vi "Main.vi"(8 "error in (no error)":errorcluster, 11 "ModuleAdmin":refnum<class "ModuleAdmin.lvclass">) -> ()   [LabVIEW 2018, in "FgenPlugins.lvlib"]
uses:
  FgenPlugins.lvlib
  <userlib>/NIST/ModuleAdminLib/ModuleAdmin/ModuleAdmin.lvclass
  C:/Program Files (x86)/National Instruments/LabVIEW 2018/user.lib/NIST/ModuleAdminLib/ModuleAdminBase/ModuleAdminBase.lvclass
  FgenShared/clStopArgument.ctl
  FgenPluginBaseClass/FgenPluginsBase.lvclass
  C:/Program Files (x86)/National Instruments/LabVIEW 2018/user.lib/NIST/BaseClasses/BasePlugin_class/BasePlugin.lvclass
  <userlib>/NIST/ModuleAdminLib/ModuleAdmin/ModuleAdmin.lvclass/ModuleAdmin.ctl
  FgenPluginBaseClass/FgenPluginsBase.lvclass/FgenPluginsBase.ctl
  MemberClasses/FunctionBaseClass/FunctionBase.lvclass/FunctionBase.ctl
  TypeDefs/clTriggers.ctl
  TypeDefs/Trigger.ctl
  TypeDefs/TriggerType.ctl
  <userlib>/NIST/BaseClasses/BasePlugin_class/BasePlugin.lvclass/BasePlugin.ctl
  TypeDefs/InitOptions.ctl
  TypeDefs/Channels.ctl
  TypeDefs/Channel.ctl
  <vilib>/Utility/error.llb/DialogType.ctl
  <userlib>/NIST/ModuleAdminLib/ModuleAdmin/Accessors/Read ShowPanel_.vi
  <userlib>/NIST/ModuleAdminLib/ModuleAdmin/Accessors/Write ShowPanel_.vi
  FgenPluginBaseClass/Accessors/Read FunctionClass.vi
  FgenPluginBaseClass/Accessors/Write FunctionClass.vi
  MemberClasses/FunctionBaseClass/Accessors/Write Waveforms.vi
  MemberClasses/FunctionBaseClass/Accessors/Read Waveforms.vi
  FgenPluginBaseClass/Accessors/Write Triggers.vi
  FgenPluginBaseClass/Read Triggers.vi
  <userlib>/NIST/BaseClasses/BasePlugin_class/Accessors/Read PluginIniFilePath.vi
  <userlib>/NIST/ModuleAdminLib/ModuleAdmin/Accessors/Read CloneRegRef.vi
  <extravilib>/ChannelInstances/Tag-bool/Read With Abort.vi
  <extravilib>/ChannelInstances/Tag-bool/Write With Abort.vi
  <extravilib>/ChannelInstances/Tag-bool/Instantiate.vi
  <extravilib>/ChannelInstances/Tag-bool/EndpointRead.vi
  <vilib>/Utility/error.llb/Error Cluster From Error Code.vi
  <extravilib>/ChannelInstances/Tag-bool/Endpoint.vi
  <vilib>/ErrorRing/Error Ring.xnode
  MemberClasses/FunctionBaseClass/FunctionBase.lvclass
  <userlib>/NIST/ModuleAdminLib/CloneRegistration/CloneRegistration.lvclass
  FgenShared/FgenShared.lvlib
  <userlib>/NIST/BaseClasses/Object_class/BaseObject.lvclass
  <userlib>/NIST/ModuleAdminLib/ModuleAdmin.lvlib
  <extravilib>/ChannelInstances/Tag-bool.lvlib
panel:
  out "Class Name":string
  out "INI File Name":string
  out "error out":errorcluster
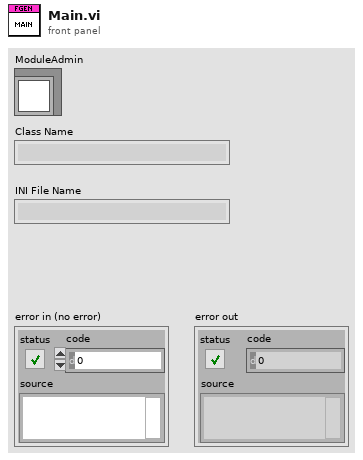
[diagram p1: front panel]
types:
  T1 = typedef "FgenShared.lvlib/clRequestEvents.ctl" = cluster{"StopRequest":refnum<user-event>, "PathToINI":refnum<user-event>, " LoadPlugin":refnum<user-event>, "ShowPanel":refnum<user-event>, "Initialize":refnum<user-event>, "GetChannels":refnum<user-event>, "SetChannels":refnum<user-event>, "Abort":refnum<user-event>, "Initiate":refnum<user-event>, "ConfigDlg":refnum<user-event>, "GetFunction":refnum<user-event>, "SetFunction":refnum<user-event>, "ConfigFunction":refnum<user-event>, "GetWfrm":refnum<user-event>, "SetWfrm":refnum<user-event>, "GetTriggers":refnum<user-event>, "SetTriggers":refnum<user-event>, "ConfigTriggers":refnum<user-event>, "Close":refnum<user-event>, "GetFunctionParams":refnum<user-event>, "SetFunctionParams":refnum<user-event>, "GetFunctionArbs":refnum<user-event>, "SetFunctionArbs":refnum<user-event>, "GetFunctionSampleRate":refnum<user-event>, "SetFunctionSampleRate":refnum<user-event>}
  T2 = typedef "FgenShared.lvlib/clBroadcastEvents.ctl" = cluster{"DidInit":refnum<user-event>, "StatusUpdate":refnum<user-event>, "ErrorReport":refnum<user-event>, "DidStop":refnum<user-event>, "PathToINI":refnum<user-event>, "Channels":refnum<user-event>, "Function":refnum<user-event>, "Waveforms":refnum<user-event>, "Triggers":refnum<user-event>, "FunctionParams":refnum<user-event>, "FunctionArbs":refnum<user-event>, "FunctionSampleRate":refnum<user-event>}
  T3 = typedef "FgenShared.lvlib/clStopArgument.ctl" = cluster{"Exit via Stop Module Req?":bool, "Wait for Module to stop?":bool, "ModuleAdmin":refnum<class "ModuleAdmin.lvclass">}
  T4 = enum32{"Invalid", "Standard", "Closed", "Hidden", "Minimized", "Maximized"}
  T5 = typedef "FgenPlugins.lvlib/clTriggers.ctl" = cluster{"Count":i32, "Triggers":T6[]}
  T6 = typedef "FgenPlugins.lvlib/Trigger.ctl" = cluster{"Source":string, "Slope":enum16{"Positive", "Negative", "Either"}, "Threshold":dbl, "Delay":dbl, "TriggerType":T7}
  T7 = typedef "FgenPlugins.lvlib/TriggerType.ctl" = enum16{"None", "Start", "Stop", "Hold", "Resume", "Advance"}
  T8 = typedef "FgenPlugins.lvlib/InitOptions.ctl" = cluster{"IDQuery":bool, "Reset":bool}
  T9 = typedef "FgenPlugins.lvlib/Channels.ctl" = cluster{"Count":u16, "Channel":T10[]}
  T10 = typedef "FgenPlugins.lvlib/Channel.ctl" = cluster{"Name":string, "Enabled":bool, "Operation":enum16{"Continuous", "Burst"}, "Impedance (50)":dbl, "Handle":string, "Connected":bool, "Mode (Function)":enum16{"Function", "Arbitrary", "Sequence"}}
  T11 = typedef "Tag-bool.lvlib/))Channel.ctl" = refnum<queue>
  T12 = typedef "DialogType.ctl" = u16
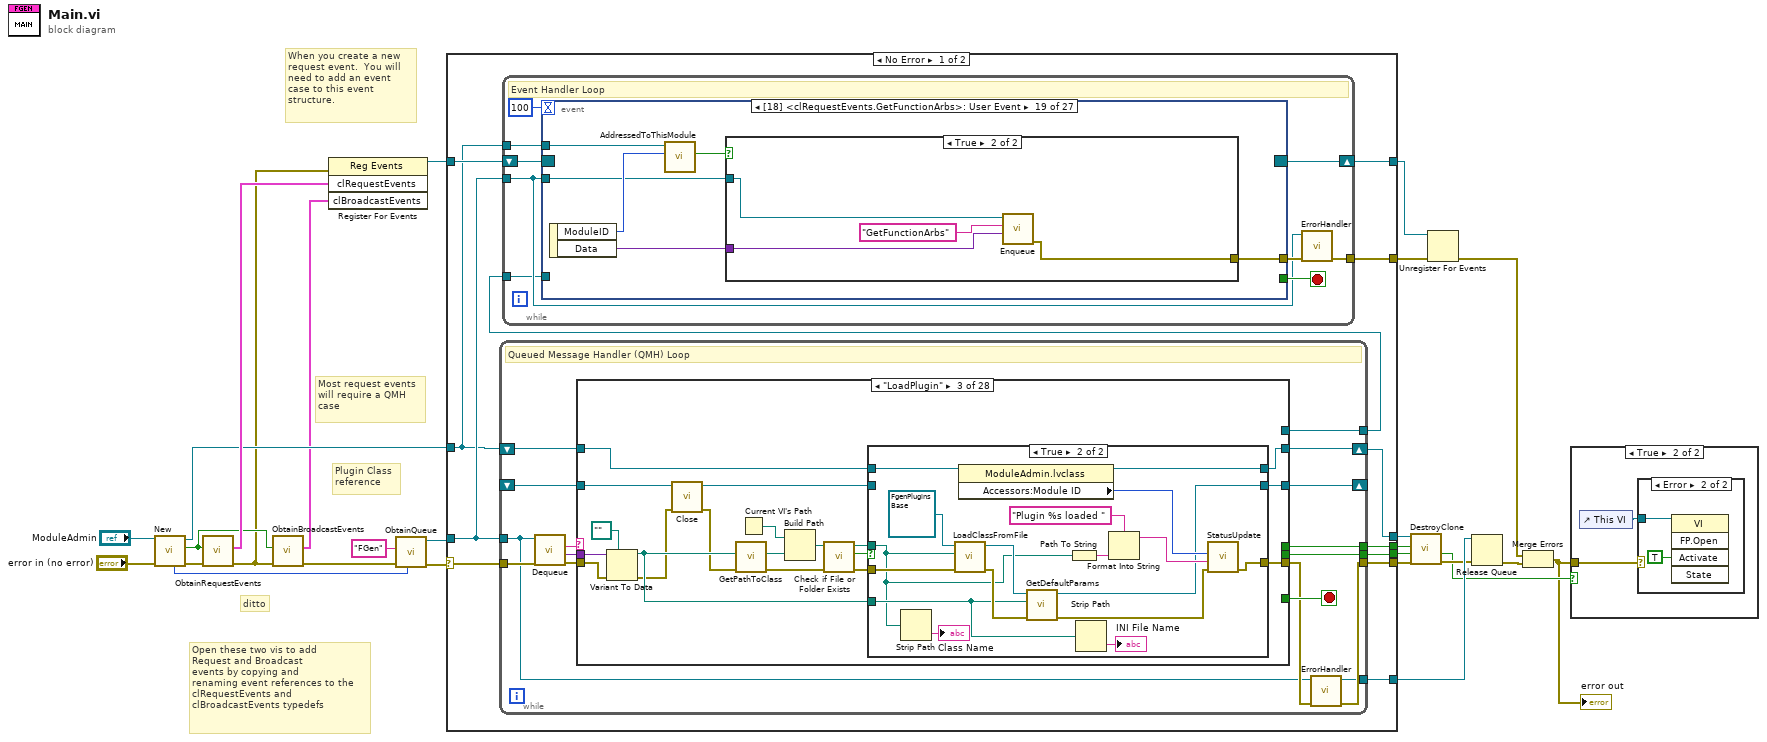
[diagram p0: block diagram]
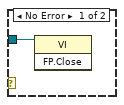
[diagram p3: hidden frame]
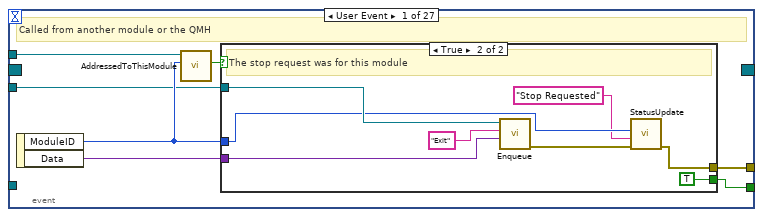
[diagram p4: hidden frame]
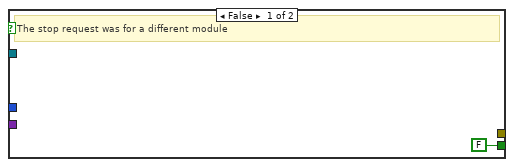
[diagram p5: hidden frame]
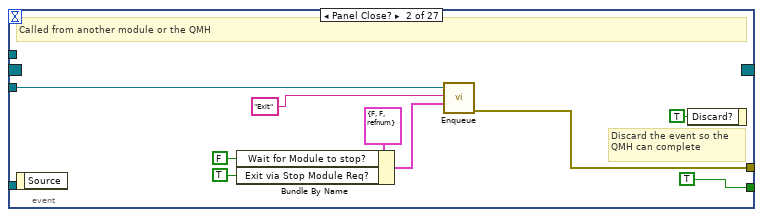
[diagram p6: hidden frame]
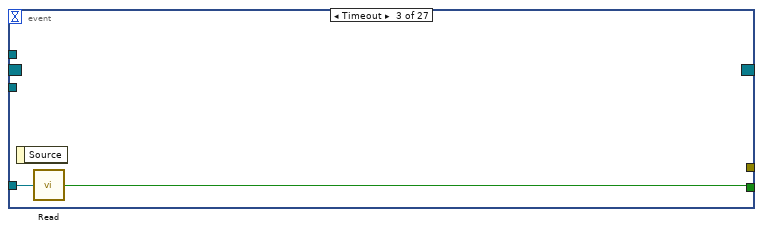
[diagram p7: hidden frame]
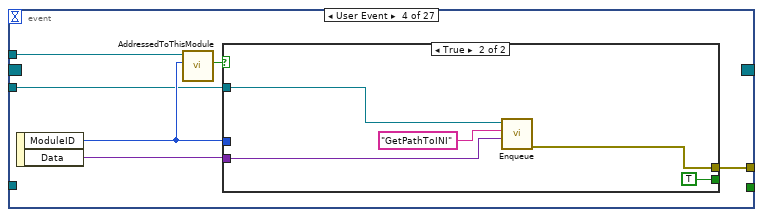
[diagram p8: hidden frame]
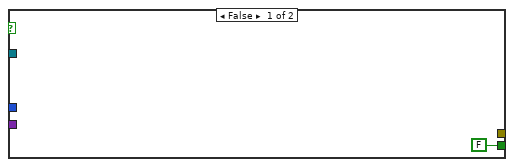
[diagram p9: hidden frame]
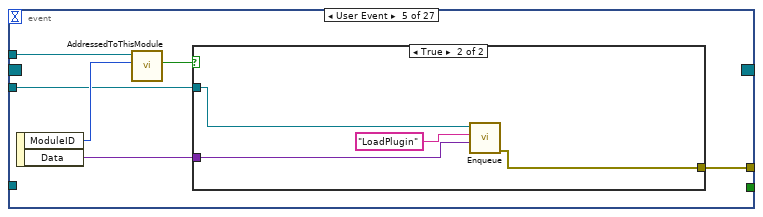
[diagram p10: hidden frame]
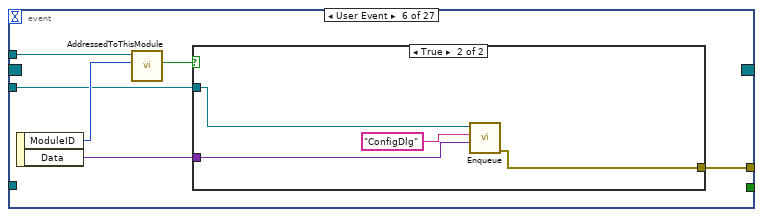
[diagram p12: hidden frame]
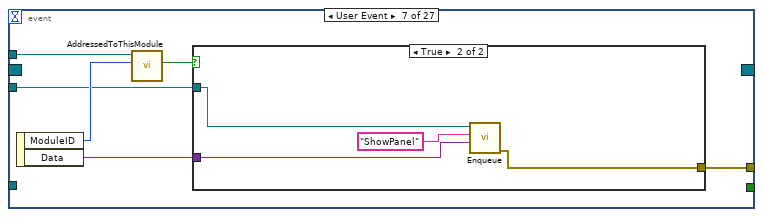
[diagram p14: hidden frame]
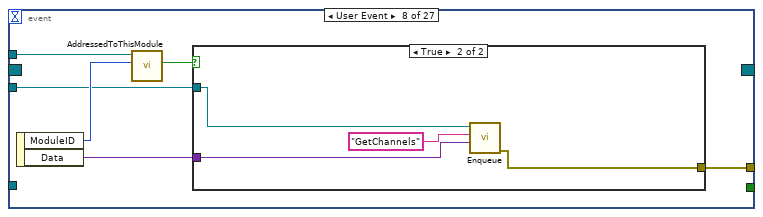
[diagram p16: hidden frame]
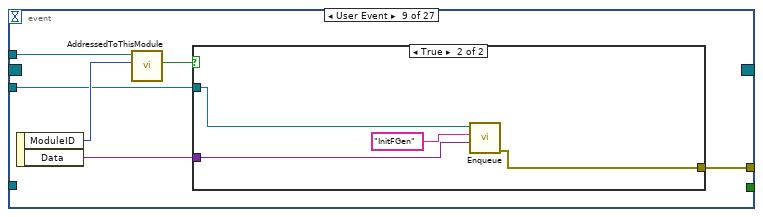
[diagram p18: hidden frame]
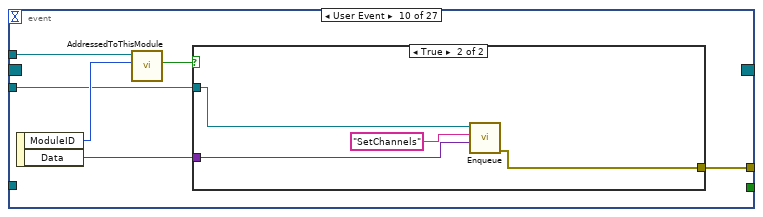
[diagram p20: hidden frame]
diagram:
  # "Plugin Class\nreference"
  # "Open these two vis to add\nRequest and Broadcast \nevents by copying and \nrenaming event references to the \nclRequestEvents and \nclBroadcastEvents typedefs"
  # "ditto"
  # "Most request events\nwill require a QMH\ncase"
  # "When you create a new request event.  You will need to add an event case to this event structure."
  n1 = call <userlib>:"New.vi"("error in (no error)"="error in (no error)", "ModuleAdmin"="ModuleAdmin") -> ("error out"=w24:errorcluster, "First?"=w17:bool, "ModuleAdmin"=w20:refnum<class "ModuleAdmin.lvclass">, "Module ID"=w6:i32)  [unwired: 6 in]
  n2 = call "ObtainRequestEvents.vi"("error in (no error)"=w24, "CreateNew (F)"=w17) -> ("error out"=w16:errorcluster, "clRequestEvents"=w23:T1)  [unwired: 8 in]
  n3 = call "ObtainBroadcastEvents.vi"("error in (no error)"=w16, "CreateNew? (F)"=w17) -> ("error out"=w18:errorcluster, "clBroadcastEvents"=w15:T2)  [unwired: 8 in]
  n4 = register-events(error in=w16, w23, w15) -> (reference out=w14:refnum<event-registration>)  [unwired: 1 in, 1 out]
  n5 = call "ObtainQueue.vi"("Module ID"=w6, "error in (no error)"=w18, "ModuleName"="FGen") -> ("error out"=w22:errorcluster, "MessageQueue"=w21:refnum<queue>)  [unwired: 7 in]
  n6 = case shown="No Error" w22 {
    selector: w22 -> [w38 w761]
    tunnel: w21 -> [w36 w758]
    tunnel: w20 -> [w33 w759]
    tunnel: [w37 w753] -> w13
    tunnel: [w35 w758] -> w19
    tunnel: w14 -> [w34 w754]
    tunnel: [w32 w757] -> w11
    tunnel: [w31 _] -> w10
    tunnel: [w30 _] -> w9
    tunnel: [w29 w753] -> w4
    tunnel: [w27 w754] -> w3
    frame No Error {
      n7 = while {
        tunnel: w36 -> [w318]
        tunnel: w38 -> [w331]
        tunnel: [w324] -> w37
        tunnel: [w317] -> w35
        tunnel: [w326] -> w31
        tunnel: [w325] -> w30
        shift-right: [w322] -> _
        shift-left: _ -> [w321]
        shift-right: [w320] -> w32
        shift-left: w33 -> [w327]
        tunnel: [w319] -> w28
        stop <- w332 stop-if-true
        # "Queued Message Handler (QMH) Loop"
        n8 = call "Dequeue.vi"("error in (no error)"=w331, "MessageQueue"=w318) -> ("error out"=w330:errorcluster, "Message Data"=w328:variant, "Message"=w329:string)  [unwired: 6 in, 1 out]
        n9 = case shown="\"LoadPlugin\"" w329 {
          selector: w329 -> [_ _ _ _ _ _ _ _ _ _ _ _ _ _ _ _ _ _ _ _ _ _ _ _ _ _ _ w741]
          tunnel: [_ _ _ _ _ _ _ _ _ _ _ _ _ _ _ _ _ _ _ _ _ _ _ _ _ w719 _ _] -> w332
          tunnel: w327 -> [w353 w370 w381 w430 w444 w451 w481 w499 w510 w521 w536 w551 w566 w584 w595 w607 w617 w624 w633 w650 w665 w672 w680 w689 w700 w713 w722 w744]
          tunnel: [w342 w363 w382 w424 w442 w447 w472 w494 w501 w515 w533 w548 w563 w573 w593 w598 w611 w619 w634 w643 w656 w666 w677 w686 w701 w718 w723 w740] -> w323
          tunnel: w330 -> [_ w373 w390 w429 w438 w457 w479 w497 w508 w519 w527 w542 w557 w580 w591 w606 w613 w625 w629 w652 w662 w674 w682 w691 w695 w709 w731 _]
          tunnel: w328 -> [_ w372 w392 _ _ w452 _ _ _ _ w529 w544 w559 w579 _ w605 _ _ _ w651 w663 _ _ _ _ w717 w730 _]
          tunnel: [_ _ _ _ _ _ _ _ _ _ _ _ _ _ _ _ _ _ _ _ _ _ _ _ _ w715 _ _] -> w326
          tunnel: [_ _ _ _ _ _ _ _ _ _ _ _ _ _ _ _ _ _ _ _ _ _ _ _ _ w714 _ _] -> w325
          tunnel: [refnum<class "FgenPluginsBase.lvclass"> refnum ("MyPlugins.lvlib:MyPluginsBase.lvclass") w362 w380 w427 w437 w446 w471 w493 w506 w517 w523 w538 w553 w572 w587 w596 w609 w623 w630 w636 w660 w669 w681 w690 w698 w712 w721 w738] -> w322
          tunnel: w321 -> [_ w362 w377 w428 w439 w459 w480 w498 w509 w520 w531 w546 w561 w582 w592 w608 w615 w626 w632 w649 w661 w673 w683 w692 w699 w711 w721 w738]
          tunnel: [w333 w369 w378 w426 w443 w445 w476 w496 w507 w518 w535 w550 w565 w583 w585 w597 w610 w622 w627 w642 w655 w668 w679 w688 w697 w707 w720 w737] -> w320
          tunnel: [_ _ _ _ _ _ _ _ _ _ _ _ _ _ _ _ _ _ _ _ _ _ _ _ _ w702 _ _] -> w319
          frame "Initialize" {
            # "Initialize is always called after ObtainQueue.vi is run"
            n10 = property class="ModuleAdmin.lvclass"(reference=w353) -> (reference out=w339:refnum<class "ModuleAdmin.lvclass">, error out=w350:errorcluster, "Accessors:Module ID"=w341:i32, "Accessors:ShowPanel_"=w336:bool, "Accessors:External Launch"=w335:bool, "Accessors:ModuleName"=w337:string)  [unwired: 1 in]
            n11 = Compound Arithmetic op=OR(w336, invert w335) -> (w334:bool)
            n12 = Select(t=T4."Standard" ("Front Panel Window:State"), s=w334, f=T4."Hidden" ("Front Panel Window:State")) -> (s? t:f=w346:T4)
            n13 = invoke class="VI" method="FP.Open"(error in=w350, "State"=w346) -> (error out=w349:errorcluster)  [unwired: 3 in, 4 out]
            n14 = call <userlib>:"ModuleName.vi"("Name"=w337, "ModuleID"=w341) -> ("ModuleName"=w345:string)  [unwired: 9 in]
            n15 = property class="VI"(error in=w349, "Front Panel.Title"=w345) -> (reference out=w352:refnum<vi>, error out=w351:errorcluster)  [unwired: 1 in]
            n16 = invoke class="VI" method="FP.Center"(reference=w352, error in=w351) -> (error out=w340:errorcluster)  [unwired: 1 in, 2 out]
            n17 = case shown="True" w335 {
              tunnel: [w354 w360] -> w343
              tunnel: [w355 w357] -> w333
              tunnel: w340 -> [w354 w359]
              tunnel: w339 -> [w355 w356]
              frame False {
              }
              frame True {
                n18 = call <userlib>:"WaitOnModuleSync.vi"("error in (no error)"=w359, "ModuleAdmin"=w356) -> ("error out"=w361:errorcluster, "ModuleAdmin"=w358:refnum<class "ModuleAdmin.lvclass">)  [unwired: 8 in]
                n19 = call <userlib>:"WaitOnEventSync.vi"("error in (no error)"=w361, "ModuleAdmin"=w358) -> ("error out"=w360:errorcluster, "ModuleAdmin"=w357:refnum<class "ModuleAdmin.lvclass">)  [unwired: 8 in]
              }
            }
            n20 = call "DidInit.vi"("Init?"=TRUE, "error in (no error)"=w343, "ModuleAdmin"=w333) -> ("error out"=w342:errorcluster)  [unwired: 8 in]
          }
          frame "ShowPanel" {
            n21 = Variant To Data(error in=w373, type=TRUE, Variant=w372) -> (data=w365:bool, error out=w368:errorcluster)
            n22 = Select(t=T4."Standard" ("Front Panel Window:State"), s=w365, f=T4."Hidden" ("Front Panel Window:State")) -> (s? t:f=w364:T4)
            n23 = property class="VI"(error in=w368, "FP.State"=w364) -> (error out=w363:errorcluster)  [unwired: 1 in, 1 out]
            n24 = property class="ModuleAdmin.lvclass"(reference=w370, "Accessors:ShowPanel_"=w365) -> (reference out=w369:refnum<class "ModuleAdmin.lvclass">)  [unwired: 1 in, 1 out]
          }
          frame "LoadPlugin" {
            n25 = Variant To Data(error in=w390, type=path "", Variant=w392) -> (data=w379:path, error out=w375:errorcluster)
            n26 = call-dynamic "Close.vi"("error in (no error)"=w375, "FgenPluginsBase in"=w377) -> ("error out"=w374:errorcluster, "FgenPluginsBase out"=w376:refnum<class "FgenPluginsBase.lvclass">)  [unwired: 8 in]
            n27 = call <userlib>:"GetPathToClass.vi"("error in (no error)"=w374, "configuration file path"=w379) -> ("error IO"=w386:errorcluster, "PathToClass"=w389:path)  [unwired: 8 in]
            n28 = Current VI's Path() -> (path=w388:path)
            n29 = Build Path(base path=w388, name or relative path=w389) -> (appended path=w387:path)
            n30 = call <vilib>:"Check if File or Folder Exists.vi"("error in (no error)"=w386, "path"=w387) -> ("error out"=w383:errorcluster, "file or folder exists?"=w385:bool, "dup path"=w384:path)  [unwired: 7 in]
            n31 = case shown="True" w385 {
              tunnel: w384 -> [w396 w406]
              tunnel: w383 -> [_ w421]
              tunnel: [w395 w416] -> w382
              tunnel: w381 -> [w393 w415]
              tunnel: w376 -> [w394 _]
              tunnel: [w394 w410] -> w380
              tunnel: w379 -> [_ w407]
              tunnel: [w393 w413] -> w378
              frame False {
                n32 = Path To String(path=w396) -> (string=w397:string)
                n33 = xnode "Error Ring"("parameter 0"=w397) -> ("error out"=w395:errorcluster)
              }
              frame True {
                n34 = Strip Path(path=w406) -> (name=→"Class Name":string)  [unwired: 1 out]
                n35 = call-dynamic "LoadClassFromFile.vi"("error in (no error)"=w421, "class path"=w406, "reference in"=refnum<class "FgenPluginsBase.lvclass"> refnum ("MyPlugins.lvlib:MyPluginsBase.lvclass")) -> ("error out"=w412:errorcluster, "reference out"=w411:refnum<class "FgenPluginsBase.lvclass">)  [unwired: 7 in]
                n36 = property class="ModuleAdmin.lvclass"(reference=w415) -> (reference out=w413:refnum<class "ModuleAdmin.lvclass">, "Accessors:Module ID"=w414:i32)  [unwired: 1 in, 1 out]
                n37 = call-dynamic "GetDefaultParams.vi"("error in (no error)"=w412, "Path"=w407, "FgenPluginsBase in"=w411) -> ("error out"=w409:errorcluster, "FgenPluginsBase out"=w410:refnum<class "FgenPluginsBase.lvclass">)  [unwired: 7 in]
                n38 = Path To String(path=w406) -> (string=w418:string)
                n39 = Strip Path(path=w407) -> (name=→"INI File Name":string)  [unwired: 1 out]
                n40 = Format Into String(format string="Plugin %s loaded ", w418) -> (resulting string=w417:string)  [unwired: 2 in, 1 out]
                n41 = call "StatusUpdate.vi"("error in (no error)"=w409, "Status"=w417, "ModuleID"=w414) -> ("error out"=w416:errorcluster)  [unwired: 8 in]
              }
            }
          }
          frame "ConfigDlg" {
            n42 = call-dynamic "ConfigDlg.vi"("error in (no error)"=w429, "FgenPluginsBase in"=w428) -> ("error out"=w425:errorcluster, "Changed"=w422:bool, "FgenPluginsBase out"=w427:refnum<class "FgenPluginsBase.lvclass">)  [unwired: 7 in]
            n43 = property class="ModuleAdmin.lvclass"(reference=w430) -> (reference out=w426:refnum<class "ModuleAdmin.lvclass">, "Accessors:Module ID"=w423:i32)  [unwired: 1 in, 1 out]
            n44 = case shown="True" w422 {
              tunnel: w425 -> [w431 w435]
              tunnel: [w431 w434] -> w424
              tunnel: w423 -> [_ w433]
              frame False {
              }
              frame True {
                n45 = call "StatusUpdate.vi"("error in (no error)"=w435, "Status"="Configuration Updated", "ModuleID"=w433) -> ("error out"=w434:errorcluster)  [unwired: 8 in]
              }
            }
          }
          frame "ConfigFunction" {
            n46 = call-dynamic "ConfigFunction.vi"("error in (no error)"=w438, "FgenPluginsBase in"=w439) -> ("error out"=w436:errorcluster, "FgenPluginsBase out"=w437:refnum<class "FgenPluginsBase.lvclass">)  [unwired: 8 in]
            n47 = property class="ModuleAdmin.lvclass"(reference=w444) -> (reference out=w443:refnum<class "ModuleAdmin.lvclass">, "Accessors:Module ID"=w441:i32)  [unwired: 1 in, 1 out]
            n48 = call "StatusUpdate.vi"("error in (no error)"=w436, "Status"="Function Configured", "ModuleID"=w441) -> ("error out"=w442:errorcluster)  [unwired: 8 in]
          }
          frame "SetFunction" {
            n49 = property class="FgenPluginsBase.lvclass"(reference=w459, error in=w457) -> (reference out=w458:refnum<class "FgenPluginsBase.lvclass">, error out=w455:errorcluster, "Accessors:FunctionClass"=w456:refnum<class "FunctionBase.lvclass">)
            n50 = disable-structure shown="Enabled" {
              disable-tunnel: w456 -> [w464 w468]
              disable-tunnel: w455 -> [w463 w467]
              disable-tunnel: [w462 w466] -> w454
              disable-tunnel: [w461 w465] -> w453
              disable-tunnel: w452 -> [w460 w469]
              frame Disabled {
                n51 = call-dynamic "SetConfig.vi"("error in (no error)"=w463, "Variant"=w460, "FunctionBase in"=w464) -> ("error out"=w462:errorcluster, "FunctionBase out"=w461:refnum<class "FunctionBase.lvclass">)  [unwired: 7 in]
              }
              frame Enabled {
                n52 = Variant To Data(error in=w467, type=w468, Variant=w469) -> (data=w465:refnum<class "FunctionBase.lvclass">, error out=w466:errorcluster)
              }
            }
            n53 = property class="FgenPluginsBase.lvclass"(reference=w458, error in=w454, "Accessors:FunctionClass"=w453) -> (reference out=w446:refnum<class "FgenPluginsBase.lvclass">, error out=w448:errorcluster)
            n54 = property class="ModuleAdmin.lvclass"(reference=w451) -> (reference out=w445:refnum<class "ModuleAdmin.lvclass">, "Accessors:Module ID"=w449:i32)  [unwired: 1 in, 1 out]
            n55 = call "StatusUpdate.vi"("error in (no error)"=w448, "Status"="Function Set", "ModuleID"=w449) -> ("error out"=w447:errorcluster)  [unwired: 8 in]
          }
          frame "GetFunction" {
            n56 = property class="FgenPluginsBase.lvclass"(reference=w480, error in=w479) -> (reference out=w471:refnum<class "FgenPluginsBase.lvclass">, error out=w477:errorcluster, "Accessors:FunctionClass"=w478:refnum<class "FunctionBase.lvclass">)
            n57 = property class="ModuleAdmin.lvclass"(reference=w481) -> (reference out=w476:refnum<class "ModuleAdmin.lvclass">, "Accessors:Module ID"=w475:i32)  [unwired: 1 in, 1 out]
            n58 = disable-structure shown="Enabled" {
              disable-tunnel: w478 -> [w485 w487]
              disable-tunnel: w477 -> [w484 w486]
              disable-tunnel: [w483 w487] -> w474
              disable-tunnel: [w482 w486] -> w473
              frame Disabled {
                n59 = call-dynamic "GetConfig.vi"("error in (no error)"=w484, "FunctionBase in"=w485) -> ("error out"=w482:errorcluster, "Config"=w483:variant)  [unwired: 7 in, 1 out]
              }
              frame Enabled {
              }
            }
            n60 = To Variant(anything=w474) -> (Variant=w470:variant)
            n61 = call "Function.vi"("ModuleID"=w475, "error in (no error)"=w473, "Function"=w470) -> ("error out"=w472:errorcluster)  [unwired: 8 in]
          }
          frame "GetFunctionParams" {
            n62 = property class="FgenPluginsBase.lvclass"(reference=w498, error in=w497) -> (reference out=w493:refnum<class "FgenPluginsBase.lvclass">, error out=w490:errorcluster, "Accessors:FunctionClass"=w489:refnum<class "FunctionBase.lvclass">)
            n63 = property class="ModuleAdmin.lvclass"(reference=w499) -> (reference out=w496:refnum<class "ModuleAdmin.lvclass">, "Accessors:Module ID"=w495:i32)  [unwired: 1 in, 1 out]
            n64 = call-dynamic "GetSignalParams.vi"("error in (no error)"=w490, "FunctionBase in"=w489) -> ("error out"=w491:errorcluster, "Params"=w488:variant)  [unwired: 7 in, 1 out]
            n65 = To Variant(anything=w488) -> (Variant=w492:variant)
            n66 = call "FunctionParams.vi"("ModuleID"=w495, "error in (no error)"=w491, "Function"=w492) -> ("error out"=w494:errorcluster)  [unwired: 8 in]
          }
          frame "GetFunctionArbs" {
            n67 = property class="FgenPluginsBase.lvclass"(reference=w509, error in=w508) -> (reference out=w506:refnum<class "FgenPluginsBase.lvclass">, error out=w505:errorcluster, "Accessors:FunctionClass"=w504:refnum<class "FunctionBase.lvclass">)
            n68 = property class="ModuleAdmin.lvclass"(reference=w510) -> (reference out=w507:refnum<class "ModuleAdmin.lvclass">, "Accessors:Module ID"=w503:i32)  [unwired: 1 in, 1 out]
            n69 = call-dynamic "GetFunctionConfig.vi"("error in (no error)"=w505, "FunctionBase In"=w504) -> ("error out"=w502:errorcluster, "FunctionConfig"=w500:variant)  [unwired: 7 in, 1 out]
            n70 = call "FunctionArbs.vi"("ModuleID"=w503, "error in (no error)"=w502, "Function"=w500) -> ("error out"=w501:errorcluster)  [unwired: 8 in]
          }
          frame "GetFunctionSampleRate" {
            n71 = property class="FgenPluginsBase.lvclass"(reference=w520, error in=w519) -> (reference out=w517:refnum<class "FgenPluginsBase.lvclass">, error out=w514:errorcluster, "Accessors:FunctionClass"=w513:refnum<class "FunctionBase.lvclass">)
            n72 = property class="ModuleAdmin.lvclass"(reference=w521) -> (reference out=w518:refnum<class "ModuleAdmin.lvclass">, "Accessors:Module ID"=w516:i32)  [unwired: 1 in, 1 out]
            n73 = call-dynamic "GetFunctionSampleRate.vi"("error in (no error)"=w514, "FunctionBase in"=w513) -> ("error out"=w511:errorcluster, "SampleRate"=w512:variant)  [unwired: 7 in, 1 out]
            n74 = call "FunctionSampleRate.vi"("ModuleID"=w516, "error in (no error)"=w511, "SampleRate"=w512) -> ("error out"=w515:errorcluster)  [unwired: 8 in]
          }
          frame "SetFunctionParams" {
            n75 = property class="FgenPluginsBase.lvclass"(reference=w531, error in=w527) -> (reference out=w528:refnum<class "FgenPluginsBase.lvclass">, error out=w526:errorcluster, "Accessors:FunctionClass"=w530:refnum<class "FunctionBase.lvclass">)
            n76 = call-dynamic "SetSignalParams.vi"("error in (no error)"=w526, "Variant"=w529, "FunctionBase in"=w530) -> ("error out"=w524:errorcluster, "FunctionBase out"=w525:refnum<class "FunctionBase.lvclass">)  [unwired: 7 in]
            n77 = property class="FgenPluginsBase.lvclass"(reference=w528, error in=w524, "Accessors:FunctionClass"=w525) -> (reference out=w523:refnum<class "FgenPluginsBase.lvclass">, error out=w522:errorcluster)
            n78 = property class="ModuleAdmin.lvclass"(reference=w536) -> (reference out=w535:refnum<class "ModuleAdmin.lvclass">, "Accessors:Module ID"=w534:i32)  [unwired: 1 in, 1 out]
            n79 = call "StatusUpdate.vi"("error in (no error)"=w522, "Status"="FunctionParams Set", "ModuleID"=w534) -> ("error out"=w533:errorcluster)  [unwired: 8 in]
          }
          frame "SetFunctionArbs" {
            n80 = property class="FgenPluginsBase.lvclass"(reference=w546, error in=w542) -> (reference out=w543:refnum<class "FgenPluginsBase.lvclass">, error out=w541:errorcluster, "Accessors:FunctionClass"=w545:refnum<class "FunctionBase.lvclass">)
            n81 = call-dynamic "SetFunctionArbs.vi"("error in (no error)"=w541, "Variant"=w544, "FunctionBase in"=w545) -> ("error out"=w539:errorcluster, "FunctionBase out"=w540:refnum<class "FunctionBase.lvclass">)  [unwired: 7 in]
            n82 = property class="FgenPluginsBase.lvclass"(reference=w543, error in=w539, "Accessors:FunctionClass"=w540) -> (reference out=w538:refnum<class "FgenPluginsBase.lvclass">, error out=w537:errorcluster)
            n83 = property class="ModuleAdmin.lvclass"(reference=w551) -> (reference out=w550:refnum<class "ModuleAdmin.lvclass">, "Accessors:Module ID"=w549:i32)  [unwired: 1 in, 1 out]
            n84 = call "StatusUpdate.vi"("error in (no error)"=w537, "Status"="FunctionConfig Set", "ModuleID"=w549) -> ("error out"=w548:errorcluster)  [unwired: 8 in]
          }
          frame "SetFunctionSampleRate" {
            n85 = property class="FgenPluginsBase.lvclass"(reference=w561, error in=w557) -> (reference out=w558:refnum<class "FgenPluginsBase.lvclass">, error out=w556:errorcluster, "Accessors:FunctionClass"=w560:refnum<class "FunctionBase.lvclass">)
            n86 = call-dynamic "SetFunctionSampleRate.vi"("error in (no error)"=w556, "SampleRate"=w559, "FunctionBase in"=w560) -> ("error out"=w554:errorcluster, "FunctionBase out"=w555:refnum<class "FunctionBase.lvclass">)  [unwired: 7 in]
            n87 = property class="FgenPluginsBase.lvclass"(reference=w558, error in=w554, "Accessors:FunctionClass"=w555) -> (reference out=w553:refnum<class "FgenPluginsBase.lvclass">, error out=w552:errorcluster)
            n88 = property class="ModuleAdmin.lvclass"(reference=w566) -> (reference out=w565:refnum<class "ModuleAdmin.lvclass">, "Accessors:Module ID"=w564:i32)  [unwired: 1 in, 1 out]
            n89 = call "StatusUpdate.vi"("error in (no error)"=w552, "Status"="FunctionSampleRate Set", "ModuleID"=w564) -> ("error out"=w563:errorcluster)  [unwired: 8 in]
          }
          frame "SetWfrm" {
            n90 = Variant To Data(error in=w580, type=waveform(dbl)[] [] ("Waveforms"), Variant=w579) -> (data=w577:waveform(dbl)[], error out=w576:errorcluster)
            n91 = property class="FgenPluginsBase.lvclass"(reference=w582, error in=w576) -> (reference out=w568:refnum<class "FgenPluginsBase.lvclass">, error out=w575:errorcluster, "Accessors:FunctionClass"=w581:refnum<class "FunctionBase.lvclass">)
            n92 = property class="FunctionBase.lvclass"(reference=w581, error in=w575, "Accessors:Waveforms"=w577) -> (reference out=w571:refnum<class "FunctionBase.lvclass">, error out=w569:errorcluster)
            n93 = property class="FgenPluginsBase.lvclass"(reference=w568, error in=w569, "Accessors:FunctionClass"=w571) -> (reference out=w572:refnum<class "FgenPluginsBase.lvclass">, error out=w567:errorcluster)
            n94 = property class="ModuleAdmin.lvclass"(reference=w584) -> (reference out=w583:refnum<class "ModuleAdmin.lvclass">, "Accessors:Module ID"=w570:i32)  [unwired: 1 in, 1 out]
            n95 = call "StatusUpdate.vi"("error in (no error)"=w567, "Status"="Waveforms Set", "ModuleID"=w570) -> ("error out"=w573:errorcluster)  [unwired: 8 in]
          }
          frame "GetWfrm" {
            n96 = property class="FgenPluginsBase.lvclass"(reference=w592, error in=w591) -> (reference out=w587:refnum<class "FgenPluginsBase.lvclass">, error out=w586:errorcluster, "Accessors:FunctionClass"=w590:refnum<class "FunctionBase.lvclass">)
            n97 = property class="FunctionBase.lvclass"(reference=w590, error in=w586) -> (error out=w588:errorcluster, "Accessors:Waveforms"=w589:waveform(dbl)[])  [unwired: 1 out]
            n98 = property class="ModuleAdmin.lvclass"(reference=w595) -> (reference out=w585:refnum<class "ModuleAdmin.lvclass">, "Accessors:Module ID"=w594:i32)  [unwired: 1 in, 1 out]
            n99 = call "Waveforms.vi"("ModuleID"=w594, "error in (no error)"=w588, "Waveforms"=w589) -> ("error out"=w593:errorcluster)  [unwired: 8 in]
          }
          frame "SetTriggers" {
            n100 = Variant To Data(error in=w606, type=T5 {"Count"=0, "Triggers"=[]} ("Triggers"), Variant=w605) -> (data=w603:T5, error out=w602:errorcluster)
            n101 = property class="FgenPluginsBase.lvclass"(reference=w608, error in=w602, "Accessors:Triggers"=w603) -> (reference out=w596:refnum<class "FgenPluginsBase.lvclass">, error out=w599:errorcluster)
            n102 = property class="ModuleAdmin.lvclass"(reference=w607) -> (reference out=w597:refnum<class "ModuleAdmin.lvclass">, "Accessors:Module ID"=w600:i32)  [unwired: 1 in, 1 out]
            n103 = call "StatusUpdate.vi"("error in (no error)"=w599, "Status"="Triggers Updated", "ModuleID"=w600) -> ("error out"=w598:errorcluster)  [unwired: 8 in]
          }
          frame "GetTriggers" {
            n104 = property class="ModuleAdmin.lvclass"(reference=w617) -> (reference out=w610:refnum<class "ModuleAdmin.lvclass">, "Accessors:Module ID"=w616:i32)  [unwired: 1 in, 1 out]
            n105 = property class="FgenPluginsBase.lvclass"(reference=w615, error in=w613) -> (reference out=w609:refnum<class "FgenPluginsBase.lvclass">, error out=w612:errorcluster, "Accessors:Triggers"=w614:T5)
            n106 = call "Triggers.vi"("ModuleID"=w616, "error in (no error)"=w612, "Triggers"=w614) -> ("error out"=w611:errorcluster)  [unwired: 8 in]
          }
          frame "ConfigTriggers" {
            n107 = property class="ModuleAdmin.lvclass"(reference=w624) -> (reference out=w622:refnum<class "ModuleAdmin.lvclass">, "Accessors:Module ID"=w618:i32)  [unwired: 1 in, 1 out]
            n108 = call-dynamic "ConfigTriggers.vi"("error in (no error)"=w625, "FgenPluginsBase in"=w626) -> ("error out"=w620:errorcluster, "FgenPluginsBase out"=w623:refnum<class "FgenPluginsBase.lvclass">)  [unwired: 8 in]
            n109 = call "StatusUpdate.vi"("error in (no error)"=w620, "Status"="Triggers Configured", "ModuleID"=w618) -> ("error out"=w619:errorcluster)  [unwired: 8 in]
          }
          frame "GetPathToINI" {
            n110 = property class="FgenPluginsBase.lvclass"(reference=w632, error in=w629) -> (reference out=w630:refnum<class "FgenPluginsBase.lvclass">, error out=w628:errorcluster, "Accessors:PluginIniFilePath"=w631:path)
            n111 = property class="ModuleAdmin.lvclass"(reference=w633) -> (reference out=w627:refnum<class "ModuleAdmin.lvclass">, "Accessors:Module ID"=w635:i32)  [unwired: 1 in, 1 out]
            n112 = call "PathToINIBroadcast.vi"("error in (no error)"=w628, "PathToINI"=w631, "ModuleID"=w635) -> ("error out"=w634:errorcluster)  [unwired: 8 in]
          }
          frame "InitFGen" {
            n113 = Variant To Data(error in=w652, type=T8 {"IDQuery"=FALSE, "Reset"=FALSE} ("InitOptions"), Variant=w651) -> (data=w647:T8, error out=w644:errorcluster)
            n114 = Unbundle By Name(w647) -> ("IDQuery"=w646:bool, "Reset"=w645:bool)
            n115 = call-dynamic "Initialize.vi"("error in (no error)"=w644, "Reset (F)"=w645, "IdQuery (F)"=w646, "FgenPluginsBase in"=w649) -> ("error out"=w639:errorcluster, "FgenPluginsBase out"=w638:refnum<class "FgenPluginsBase.lvclass">)  [unwired: 6 in]
            n116 = call-dynamic "ConfigClock.vi"("error in (no error)"=w639, "FgenPluginsBase in"=w638) -> ("error out"=w637:errorcluster, "FgenPluginsBase out"=w636:refnum<class "FgenPluginsBase.lvclass">)  [unwired: 8 in]
            n117 = property class="ModuleAdmin.lvclass"(reference=w650) -> (reference out=w642:refnum<class "ModuleAdmin.lvclass">, "Accessors:Module ID"=w641:i32)  [unwired: 1 in, 1 out]
            n118 = call "StatusUpdate.vi"("error in (no error)"=w637, "Status"="Device Initialized", "ModuleID"=w641) -> ("error out"=w643:errorcluster)  [unwired: 8 in]
          }
          frame "SetChannels" {
            n119 = Variant To Data(error in=w662, type=T9 {"Count"=0, "Channel"=[]} ("Channels"), Variant=w663) -> (data=w658:T9, error out=w659:errorcluster)
            n120 = call-dynamic "SetChannels.vi"("error in (no error)"=w659, "Channels"=w658, "FgenPluginsBase in"=w661) -> ("error out"=w657:errorcluster, "FgenPluginsBase out"=w660:refnum<class "FgenPluginsBase.lvclass">)  [unwired: 7 in]
            n121 = property class="ModuleAdmin.lvclass"(reference=w665) -> (reference out=w655:refnum<class "ModuleAdmin.lvclass">, "Accessors:Module ID"=w654:i32)  [unwired: 1 in, 1 out]
            n122 = call "StatusUpdate.vi"("error in (no error)"=w657, "Status"="Channels Updated", "ModuleID"=w654) -> ("error out"=w656:errorcluster)  [unwired: 8 in]
          }
          frame "InitGen" {
            n123 = call-dynamic "InitiateGeneration.vi"("error in (no error)"=w674, "FgenPluginsBase in"=w673) -> ("error out"=w671:errorcluster, "FgenPluginsBase out"=w669:refnum<class "FgenPluginsBase.lvclass">)  [unwired: 8 in]
            n124 = property class="ModuleAdmin.lvclass"(reference=w672) -> (reference out=w668:refnum<class "ModuleAdmin.lvclass">, "Accessors:Module ID"=w670:i32)  [unwired: 1 in, 1 out]
            n125 = call "StatusUpdate.vi"("error in (no error)"=w671, "Status"="Initiate Generation", "ModuleID"=w670) -> ("error out"=w666:errorcluster)  [unwired: 8 in]
          }
          frame "AbortGen" {
            n126 = call-dynamic "AbortGeneration.vi"("error in (no error)"=w682, "FgenPluginsBase in"=w683) -> ("error out"=w678:errorcluster, "FgenPluginsBase out"=w681:refnum<class "FgenPluginsBase.lvclass">)  [unwired: 8 in]
            n127 = property class="ModuleAdmin.lvclass"(reference=w680) -> (reference out=w679:refnum<class "ModuleAdmin.lvclass">, "Accessors:Module ID"=w676:i32)  [unwired: 1 in, 1 out]
            n128 = call "StatusUpdate.vi"("error in (no error)"=w678, "Status"="Abort Generation", "ModuleID"=w676) -> ("error out"=w677:errorcluster)  [unwired: 8 in]
          }
          frame "Close" {
            n129 = call-dynamic "Close.vi"("error in (no error)"=w691, "FgenPluginsBase in"=w692) -> ("error out"=w687:errorcluster, "FgenPluginsBase out"=w690:refnum<class "FgenPluginsBase.lvclass">)  [unwired: 8 in]
            n130 = property class="ModuleAdmin.lvclass"(reference=w689) -> (reference out=w688:refnum<class "ModuleAdmin.lvclass">, "Accessors:Module ID"=w685:i32)  [unwired: 1 in, 1 out]
            n131 = call "StatusUpdate.vi"("error in (no error)"=w687, "Status"="Closed", "ModuleID"=w685) -> ("error out"=w686:errorcluster)  [unwired: 8 in]
          }
          frame "GetChannels" {
            n132 = property class="ModuleAdmin.lvclass"(reference=w700) -> (reference out=w697:refnum<class "ModuleAdmin.lvclass">, "Accessors:Module ID"=w696:i32)  [unwired: 1 in, 1 out]
            n133 = call-dynamic "GetChannels.vi"("error in (no error)"=w695, "FgenPluginsBase in"=w699) -> ("error out"=w694:errorcluster, "Channels"=w693:cluster{"Count":u16, "Channel":T10[]}, "FgenPluginsBase out"=w698:refnum<class "FgenPluginsBase.lvclass">)  [unwired: 7 in]
            n134 = call "Channels.vi"("ModuleID"=w696, "error in (no error)"=w694, "Channels"=w693) -> ("error out"=w701:errorcluster)  [unwired: 8 in]
          }
          frame "Exit" {
            w719 = TRUE
            # "Called by the StopRequest event handler case"
            n135 = property class="ModuleAdmin.lvclass"(reference=w713) -> (reference out=w707:refnum<class "ModuleAdmin.lvclass">, "Accessors:Module ID"=w706:i32)  [unwired: 1 in, 1 out]
            n136 = call-dynamic "AbortGeneration.vi"("error in (no error)"=w709, "FgenPluginsBase in"=w711) -> ("error out"=w708:errorcluster, "FgenPluginsBase out"=w710:refnum<class "FgenPluginsBase.lvclass">)  [unwired: 8 in]
            n137 = call-dynamic "Close.vi"("error in (no error)"=w708, "FgenPluginsBase in"=w710) -> ("error out"=w704:errorcluster, "FgenPluginsBase out"=w712:refnum<class "FgenPluginsBase.lvclass">)  [unwired: 8 in]
            n138 = call "StatusUpdate.vi"("error in (no error)"=w704, "Status"="Exiting", "ModuleID"=w706) -> ("error out"=w703:errorcluster)  [unwired: 8 in]
            n139 = control-ref of="This VI"() -> (w716:refnum<vi>)
            n140 = call "HandleExit.vi"("error in (no error)"=w703, "VI Refnum"=w716, "StopArgument"=w717, "ModuleAdmin"=w707) -> ("error out"=w718:errorcluster, "Exit via Stop Module Req?"=w714:bool, "WaitForStop?"=w715:bool)  [unwired: 5 in]
            n141 = call <extravilib>:"Write.vi"("element"=w719) -> ("channel"=w702:T11)  [unwired: 1 out]
          }
          frame "Error" {
            n142 = property class="ModuleAdmin.lvclass"(reference=w722) -> (reference out=w720:refnum<class "ModuleAdmin.lvclass">, "Accessors:External Launch"=w726:bool, "Accessors:Module ID"=w724:i32)  [unwired: 1 in, 1 out]
            n143 = Variant To Data(error in=w731, type=errorcluster {"status"=FALSE, "code"=0, "source"=""} ("error constant"), Variant=w730) -> (data=w725:errorcluster, error out=w728:errorcluster)
            n144 = call "ReportError.vi"("error in (no error)"=w728, "ErrorReported"=w725, "ModuleID"=w724) -> ("error out"=w727:errorcluster)  [unwired: 8 in]
            n145 = case shown="True" w726 {
              tunnel: w727 -> [w735 w736]
              tunnel: w725 -> [w734 _]
              tunnel: [w733 w736] -> w723
              tunnel: w722 -> [w732 _]
              frame False {
                # "Todo:  Add an event to ask the user\nIf the module should stop or continue"
                # "Stand alone: now, force an exit"
                n146 = call <vilib>:"Simple Error Handler.vi"("error in (no error)"=w734) -> ()  [unwired: 4 in, 5 out]
                n147 = call "StopRequest.vi"("error in (no error)"=w735, "ModuleAdmin"=w732) -> ("error out"=w733:errorcluster)  [unwired: 8 in, 1 out]
              }
              frame True {
                # "Externally launched modules only broadcast the error msg"
              }
            }
          }
          frame Default {
            # "Called only if a message was queued and no QMH case was created"
            n148 = property class="ModuleAdmin.lvclass"(reference=w744) -> (reference out=w737:refnum<class "ModuleAdmin.lvclass">, "Accessors:Module ID"=w743:i32, "Accessors:ModuleName"=w739:string)  [unwired: 1 in, 1 out]
            n149 = call <userlib>:"ModuleName.vi"("Name"=w739, "ModuleID"=w743) -> ("ModuleName"=w742:string)  [unwired: 9 in]
            n150 = xnode "Error Ring"("parameter 0"=w741, "parameter 1"=w742) -> ("error out"=w740:errorcluster)
          }
        }
        n151 = call "ErrorHandler.vi"("error in (no error)"=w323, "MessageQueue"=w318) -> ("error out"=w324:errorcluster, "MessageQueue"=w317:refnum<queue>)  [unwired: 8 in]
      }
      n152 = while {
        tunnel: w36 -> [w41]
        shift-right: [w45] -> w27
        shift-left: w34 -> [w46]
        tunnel: w33 -> [w44]
        tunnel: [w42] -> w29
        tunnel: w28 -> [w39]
        stop <- w47 stop-if-true
        # "Event Handler Loop"
        n153 = event shown="[18] <clRequestEvents.GetFunctionArbs>: User Event" {
          selector: w46 -> [_ _ _ _ _ _ _ _ _ _ _ _ _ _ _ _ _ _ _ _ _ _ _ _ _ _ _]
          dyn-events: [_ _ _ _ _ _ _ _ _ _ _ _ _ _ _ _ _ _ _ _ _ _ _ _ _ _ _] -> w45
          timeout: 100 -> [_ _ _ _ _ _ _ _ _ _ _ _ _ _ _ _ _ _ _ _ _ _ _ _ _ _ _]
          tunnel: w41 -> [w51 w72 _ w77 w88 w98 w108 w118 w128 w138 w148 w158 w168 w178 w188 w198 w208 w218 w228 w238 w248 w258 w268 w278 w288 w298 w308]
          tunnel: [w50 TRUE w73 _ _ _ _ _ _ _ _ _ _ _ _ _ _ _ _ _ _ _ _ _ _ _ _] -> w47
          tunnel: w44 -> [w54 _ _ w76 w92 w102 w112 w122 w132 w142 w152 w162 w172 w182 w192 w202 w212 w222 w232 w242 w252 w262 w272 w282 w292 w302 w312]
          tunnel: [w49 w70 _ w75 w89 w99 w109 w119 w129 w139 w149 w159 w169 w179 w189 w199 w209 w219 w229 w239 w249 w259 w269 w279 w289 w299 w309] -> w43
          tunnel: w39 -> [_ _ w74 _ _ _ _ _ _ _ _ _ _ _ _ _ _ _ _ _ _ _ _ _ _ _ _]
          event User Event {
            # "Called from another module or the QMH"
            n154 = event-data() -> ("ModuleID"=w52:i32, "Data"=w48:variant)  [unwired: 1 in]
            n155 = call <userlib>:"AddressedToThisModule.vi"("ModuleID"=w52, "ModuleAdmin"=w54) -> ("AddressedToThisInstance?"=w53:bool)  [unwired: 8 in, 1 out]
            n156 = case shown="True" w53 {
              tunnel: w52 -> [_ w57]
              tunnel: w51 -> [_ w63]
              tunnel: [FALSE TRUE] -> w50
              tunnel: [_ w58] -> w49
              tunnel: w48 -> [_ w60]
              frame False {
                # "The stop request was for a different module"
              }
              frame True {
                # "The stop request was for this module"
                n157 = call "Enqueue.vi"("Message Data"=w60, "Message"="Exit", "MessageQueue"=w63) -> ("error out"=w59:errorcluster)  [unwired: 7 in, 1 out]
                n158 = call "StatusUpdate.vi"("error in (no error)"=w59, "Status"="Stop Requested", "ModuleID"=w57) -> ("error out"=w58:errorcluster)  [unwired: 8 in]
              }
            }
          }
          event Panel Close? {
            # "Discard the event so the QMH can complete"
            # "Called from another module or the QMH"
            n159 = event-data() -> ()  [unwired: 1 in, 1 out]
            n160 = Bundle By Name(cluster=T3 {"Exit via Stop Module Req?"=FALSE, "Wait for Module to stop?"=FALSE, "ModuleAdmin"=refnum} ("Stop Argument"), "Wait for Module to stop?"=FALSE, "Exit via Stop Module Req?"=TRUE) -> (w67:T3)
            n161 = call "Enqueue.vi"("Message Data"=w67, "Message"="Exit", "MessageQueue"=w72) -> ("error out"=w70:errorcluster)  [unwired: 7 in, 1 out]
            n162 = event-data("Discard?"=TRUE) -> ()  [unwired: 1 in, 1 out]
          }
          event Timeout {
            n163 = event-data() -> ()  [unwired: 1 in, 1 out]
            n164 = call <extravilib>:"Read.vi"("channel"=w74) -> ("element"=w73:bool)  [unwired: 1 in, 1 out]
          }
          event User Event {
            n165 = event-data() -> ("ModuleID"=w78:i32, "Data"=w79:variant)  [unwired: 1 in]
            n166 = call <userlib>:"AddressedToThisModule.vi"("ModuleID"=w78, "ModuleAdmin"=w76) -> ("AddressedToThisInstance?"=w80:bool)  [unwired: 8 in, 1 out]
            n167 = case shown="True" w80 {
              tunnel: w78 -> [_ _]
              tunnel: w77 -> [_ w86]
              tunnel: [FALSE TRUE] -> _
              tunnel: [_ w84] -> w75
              tunnel: w79 -> [_ w82]
              frame False {
                # "The stop request was for a different module"
              }
              frame True {
                # "The stop request was for this module"
                n168 = call "Enqueue.vi"("Message Data"=w82, "Message"="GetPathToINI", "MessageQueue"=w86) -> ("error out"=w84:errorcluster)  [unwired: 7 in, 1 out]
              }
            }
          }
          event User Event {
            n169 = event-data() -> ("ModuleID"=w91:i32, "Data"=w87:variant)  [unwired: 1 in]
            n170 = call <userlib>:"AddressedToThisModule.vi"("ModuleID"=w91, "ModuleAdmin"=w92) -> ("AddressedToThisInstance?"=w90:bool)  [unwired: 8 in, 1 out]
            n171 = case shown="True" w90 {
              tunnel: [_ w93] -> w89
              tunnel: w88 -> [_ w96]
              tunnel: w87 -> [_ w94]
              frame False {
              }
              frame True {
                n172 = call "Enqueue.vi"("Message Data"=w94, "Message"="LoadPlugin", "MessageQueue"=w96) -> ("error out"=w93:errorcluster)  [unwired: 7 in, 1 out]
              }
            }
          }
          event User Event {
            n173 = event-data() -> ("ModuleID"=w101:i32, "Data"=w97:variant)  [unwired: 1 in]
            n174 = call <userlib>:"AddressedToThisModule.vi"("ModuleID"=w101, "ModuleAdmin"=w102) -> ("AddressedToThisInstance?"=w100:bool)  [unwired: 8 in, 1 out]
            n175 = case shown="True" w100 {
              tunnel: [_ w103] -> w99
              tunnel: w98 -> [_ w106]
              tunnel: w97 -> [_ w104]
              frame False {
              }
              frame True {
                n176 = call "Enqueue.vi"("Message Data"=w104, "Message"="ConfigDlg", "MessageQueue"=w106) -> ("error out"=w103:errorcluster)  [unwired: 7 in, 1 out]
              }
            }
          }
          event User Event {
            n177 = event-data() -> ("ModuleID"=w111:i32, "Data"=w107:variant)  [unwired: 1 in]
            n178 = call <userlib>:"AddressedToThisModule.vi"("ModuleID"=w111, "ModuleAdmin"=w112) -> ("AddressedToThisInstance?"=w110:bool)  [unwired: 8 in, 1 out]
            n179 = case shown="True" w110 {
              tunnel: [_ w113] -> w109
              tunnel: w108 -> [_ w116]
              tunnel: w107 -> [_ w114]
              frame False {
              }
              frame True {
                n180 = call "Enqueue.vi"("Message Data"=w114, "Message"="ShowPanel", "MessageQueue"=w116) -> ("error out"=w113:errorcluster)  [unwired: 7 in, 1 out]
              }
            }
          }
          event User Event {
            n181 = event-data() -> ("ModuleID"=w121:i32, "Data"=w117:variant)  [unwired: 1 in]
            n182 = call <userlib>:"AddressedToThisModule.vi"("ModuleID"=w121, "ModuleAdmin"=w122) -> ("AddressedToThisInstance?"=w120:bool)  [unwired: 8 in, 1 out]
            n183 = case shown="True" w120 {
              tunnel: [_ w123] -> w119
              tunnel: w118 -> [_ w126]
              tunnel: w117 -> [_ w124]
              frame False {
              }
              frame True {
                n184 = call "Enqueue.vi"("Message Data"=w124, "Message"="GetChannels", "MessageQueue"=w126) -> ("error out"=w123:errorcluster)  [unwired: 7 in, 1 out]
              }
            }
          }
          event User Event {
            n185 = event-data() -> ("ModuleID"=w131:i32, "Data"=w127:variant)  [unwired: 1 in]
            n186 = call <userlib>:"AddressedToThisModule.vi"("ModuleID"=w131, "ModuleAdmin"=w132) -> ("AddressedToThisInstance?"=w130:bool)  [unwired: 8 in, 1 out]
            n187 = case shown="True" w130 {
              tunnel: [_ w133] -> w129
              tunnel: w128 -> [_ w136]
              tunnel: w127 -> [_ w134]
              frame False {
              }
              frame True {
                n188 = call "Enqueue.vi"("Message Data"=w134, "Message"="InitFGen", "MessageQueue"=w136) -> ("error out"=w133:errorcluster)  [unwired: 7 in, 1 out]
              }
            }
          }
          event User Event {
            n189 = event-data() -> ("ModuleID"=w141:i32, "Data"=w137:variant)  [unwired: 1 in]
            n190 = call <userlib>:"AddressedToThisModule.vi"("ModuleID"=w141, "ModuleAdmin"=w142) -> ("AddressedToThisInstance?"=w140:bool)  [unwired: 8 in, 1 out]
            n191 = case shown="True" w140 {
              tunnel: [_ w143] -> w139
              tunnel: w138 -> [_ w146]
              tunnel: w137 -> [_ w144]
              frame False {
              }
              frame True {
                n192 = call "Enqueue.vi"("Message Data"=w144, "Message"="SetChannels", "MessageQueue"=w146) -> ("error out"=w143:errorcluster)  [unwired: 7 in, 1 out]
              }
            }
          }
          event User Event {
            n193 = event-data() -> ("ModuleID"=w151:i32, "Data"=w147:variant)  [unwired: 1 in]
            n194 = call <userlib>:"AddressedToThisModule.vi"("ModuleID"=w151, "ModuleAdmin"=w152) -> ("AddressedToThisInstance?"=w150:bool)  [unwired: 8 in, 1 out]
            n195 = case shown="True" w150 {
              tunnel: [_ w153] -> w149
              tunnel: w148 -> [_ w156]
              tunnel: w147 -> [_ w154]
              frame False {
              }
              frame True {
                n196 = call "Enqueue.vi"("Message Data"=w154, "Message"="InitGen", "MessageQueue"=w156) -> ("error out"=w153:errorcluster)  [unwired: 7 in, 1 out]
              }
            }
          }
          event User Event {
            n197 = event-data() -> ("ModuleID"=w161:i32, "Data"=w157:variant)  [unwired: 1 in]
            n198 = call <userlib>:"AddressedToThisModule.vi"("ModuleID"=w161, "ModuleAdmin"=w162) -> ("AddressedToThisInstance?"=w160:bool)  [unwired: 8 in, 1 out]
            n199 = case shown="True" w160 {
              tunnel: [_ w163] -> w159
              tunnel: w158 -> [_ w166]
              tunnel: w157 -> [_ w164]
              frame False {
              }
              frame True {
                n200 = call "Enqueue.vi"("Message Data"=w164, "Message"="AbortGen", "MessageQueue"=w166) -> ("error out"=w163:errorcluster)  [unwired: 7 in, 1 out]
              }
            }
          }
          event User Event {
            n201 = event-data() -> ("ModuleID"=w171:i32, "Data"=w167:variant)  [unwired: 1 in]
            n202 = call <userlib>:"AddressedToThisModule.vi"("ModuleID"=w171, "ModuleAdmin"=w172) -> ("AddressedToThisInstance?"=w170:bool)  [unwired: 8 in, 1 out]
            n203 = case shown="True" w170 {
              tunnel: [_ w173] -> w169
              tunnel: w168 -> [_ w176]
              tunnel: w167 -> [_ w174]
              frame False {
              }
              frame True {
                n204 = call "Enqueue.vi"("Message Data"=w174, "Message"="ConfigFunction", "MessageQueue"=w176) -> ("error out"=w173:errorcluster)  [unwired: 7 in, 1 out]
              }
            }
          }
          event User Event {
            n205 = event-data() -> ("ModuleID"=w181:i32, "Data"=w177:variant)  [unwired: 1 in]
            n206 = call <userlib>:"AddressedToThisModule.vi"("ModuleID"=w181, "ModuleAdmin"=w182) -> ("AddressedToThisInstance?"=w180:bool)  [unwired: 8 in, 1 out]
            n207 = case shown="True" w180 {
              tunnel: [_ w183] -> w179
              tunnel: w178 -> [_ w186]
              tunnel: w177 -> [_ w184]
              frame False {
              }
              frame True {
                n208 = call "Enqueue.vi"("Message Data"=w184, "Message"="SetFunction", "MessageQueue"=w186) -> ("error out"=w183:errorcluster)  [unwired: 7 in, 1 out]
              }
            }
          }
          event User Event {
            n209 = event-data() -> ("ModuleID"=w191:i32, "Data"=w187:variant)  [unwired: 1 in]
            n210 = call <userlib>:"AddressedToThisModule.vi"("ModuleID"=w191, "ModuleAdmin"=w192) -> ("AddressedToThisInstance?"=w190:bool)  [unwired: 8 in, 1 out]
            n211 = case shown="True" w190 {
              tunnel: [_ w193] -> w189
              tunnel: w188 -> [_ w196]
              tunnel: w187 -> [_ w194]
              frame False {
              }
              frame True {
                n212 = call "Enqueue.vi"("Message Data"=w194, "Message"="GetFunction", "MessageQueue"=w196) -> ("error out"=w193:errorcluster)  [unwired: 7 in, 1 out]
              }
            }
          }
          event User Event {
            n213 = event-data() -> ("ModuleID"=w201:i32, "Data"=w197:variant)  [unwired: 1 in]
            n214 = call <userlib>:"AddressedToThisModule.vi"("ModuleID"=w201, "ModuleAdmin"=w202) -> ("AddressedToThisInstance?"=w200:bool)  [unwired: 8 in, 1 out]
            n215 = case shown="True" w200 {
              tunnel: [_ w203] -> w199
              tunnel: w198 -> [_ w206]
              tunnel: w197 -> [_ w204]
              frame False {
              }
              frame True {
                n216 = call "Enqueue.vi"("Message Data"=w204, "Message"="GetFunctionParams", "MessageQueue"=w206) -> ("error out"=w203:errorcluster)  [unwired: 7 in, 1 out]
              }
            }
          }
          event User Event {
            n217 = event-data() -> ("ModuleID"=w211:i32, "Data"=w207:variant)  [unwired: 1 in]
            n218 = call <userlib>:"AddressedToThisModule.vi"("ModuleID"=w211, "ModuleAdmin"=w212) -> ("AddressedToThisInstance?"=w210:bool)  [unwired: 8 in, 1 out]
            n219 = case shown="True" w210 {
              tunnel: [_ w213] -> w209
              tunnel: w208 -> [_ w216]
              tunnel: w207 -> [_ w214]
              frame False {
              }
              frame True {
                n220 = call "Enqueue.vi"("Message Data"=w214, "Message"="SetFunctionParams", "MessageQueue"=w216) -> ("error out"=w213:errorcluster)  [unwired: 7 in, 1 out]
              }
            }
          }
          event User Event {
            n221 = event-data() -> ("ModuleID"=w221:i32, "Data"=w217:variant)  [unwired: 1 in]
            n222 = call <userlib>:"AddressedToThisModule.vi"("ModuleID"=w221, "ModuleAdmin"=w222) -> ("AddressedToThisInstance?"=w220:bool)  [unwired: 8 in, 1 out]
            n223 = case shown="True" w220 {
              tunnel: [_ w223] -> w219
              tunnel: w218 -> [_ w226]
              tunnel: w217 -> [_ w224]
              frame False {
              }
              frame True {
                n224 = call "Enqueue.vi"("Message Data"=w224, "Message"="SetFunctionArbs", "MessageQueue"=w226) -> ("error out"=w223:errorcluster)  [unwired: 7 in, 1 out]
              }
            }
          }
          event User Event {
            n225 = event-data() -> ("ModuleID"=w231:i32, "Data"=w227:variant)  [unwired: 1 in]
            n226 = call <userlib>:"AddressedToThisModule.vi"("ModuleID"=w231, "ModuleAdmin"=w232) -> ("AddressedToThisInstance?"=w230:bool)  [unwired: 8 in, 1 out]
            n227 = case shown="True" w230 {
              tunnel: [_ w233] -> w229
              tunnel: w228 -> [_ w236]
              tunnel: w227 -> [_ w234]
              frame False {
              }
              frame True {
                n228 = call "Enqueue.vi"("Message Data"=w234, "Message"="GetFunctionArbs", "MessageQueue"=w236) -> ("error out"=w233:errorcluster)  [unwired: 7 in, 1 out]
              }
            }
          }
          event User Event {
            n229 = event-data() -> ("ModuleID"=w241:i32, "Data"=w237:variant)  [unwired: 1 in]
            n230 = call <userlib>:"AddressedToThisModule.vi"("ModuleID"=w241, "ModuleAdmin"=w242) -> ("AddressedToThisInstance?"=w240:bool)  [unwired: 8 in, 1 out]
            n231 = case shown="True" w240 {
              tunnel: [_ w243] -> w239
              tunnel: w238 -> [_ w246]
              tunnel: w237 -> [_ w244]
              frame False {
              }
              frame True {
                n232 = call "Enqueue.vi"("Message Data"=w244, "Message"="GetFunctionSampleRate", "MessageQueue"=w246) -> ("error out"=w243:errorcluster)  [unwired: 7 in, 1 out]
              }
            }
          }
          event User Event {
            n233 = event-data() -> ("ModuleID"=w251:i32, "Data"=w247:variant)  [unwired: 1 in]
            n234 = call <userlib>:"AddressedToThisModule.vi"("ModuleID"=w251, "ModuleAdmin"=w252) -> ("AddressedToThisInstance?"=w250:bool)  [unwired: 8 in, 1 out]
            n235 = case shown="True" w250 {
              tunnel: [_ w253] -> w249
              tunnel: w248 -> [_ w256]
              tunnel: w247 -> [_ w254]
              frame False {
              }
              frame True {
                n236 = call "Enqueue.vi"("Message Data"=w254, "Message"="SetFunctionSampleRate", "MessageQueue"=w256) -> ("error out"=w253:errorcluster)  [unwired: 7 in, 1 out]
              }
            }
          }
          event User Event {
            n237 = event-data() -> ("ModuleID"=w261:i32, "Data"=w257:variant)  [unwired: 1 in]
            n238 = call <userlib>:"AddressedToThisModule.vi"("ModuleID"=w261, "ModuleAdmin"=w262) -> ("AddressedToThisInstance?"=w260:bool)  [unwired: 8 in, 1 out]
            n239 = case shown="True" w260 {
              tunnel: [_ w263] -> w259
              tunnel: w258 -> [_ w266]
              tunnel: w257 -> [_ w264]
              frame False {
              }
              frame True {
                n240 = call "Enqueue.vi"("Message Data"=w264, "Message"="SetWfrm", "MessageQueue"=w266) -> ("error out"=w263:errorcluster)  [unwired: 7 in, 1 out]
              }
            }
          }
          event User Event {
            n241 = event-data() -> ("ModuleID"=w271:i32, "Data"=w267:variant)  [unwired: 1 in]
            n242 = call <userlib>:"AddressedToThisModule.vi"("ModuleID"=w271, "ModuleAdmin"=w272) -> ("AddressedToThisInstance?"=w270:bool)  [unwired: 8 in, 1 out]
            n243 = case shown="True" w270 {
              tunnel: [_ w273] -> w269
              tunnel: w268 -> [_ w276]
              tunnel: w267 -> [_ w274]
              frame False {
              }
              frame True {
                n244 = call "Enqueue.vi"("Message Data"=w274, "Message"="GetWfrm", "MessageQueue"=w276) -> ("error out"=w273:errorcluster)  [unwired: 7 in, 1 out]
              }
            }
          }
          event User Event {
            n245 = event-data() -> ("ModuleID"=w281:i32, "Data"=w277:variant)  [unwired: 1 in]
            n246 = call <userlib>:"AddressedToThisModule.vi"("ModuleID"=w281, "ModuleAdmin"=w282) -> ("AddressedToThisInstance?"=w280:bool)  [unwired: 8 in, 1 out]
            n247 = case shown="True" w280 {
              tunnel: [_ w283] -> w279
              tunnel: w278 -> [_ w286]
              tunnel: w277 -> [_ w284]
              frame False {
              }
              frame True {
                n248 = call "Enqueue.vi"("Message Data"=w284, "Message"="SetTriggers", "MessageQueue"=w286) -> ("error out"=w283:errorcluster)  [unwired: 7 in, 1 out]
              }
            }
          }
          event User Event {
            n249 = event-data() -> ("ModuleID"=w291:i32, "Data"=w287:variant)  [unwired: 1 in]
            n250 = call <userlib>:"AddressedToThisModule.vi"("ModuleID"=w291, "ModuleAdmin"=w292) -> ("AddressedToThisInstance?"=w290:bool)  [unwired: 8 in, 1 out]
            n251 = case shown="True" w290 {
              tunnel: [_ w293] -> w289
              tunnel: w288 -> [_ w296]
              tunnel: w287 -> [_ w294]
              frame False {
              }
              frame True {
                n252 = call "Enqueue.vi"("Message Data"=w294, "Message"="GetTriggers", "MessageQueue"=w296) -> ("error out"=w293:errorcluster)  [unwired: 7 in, 1 out]
              }
            }
          }
          event User Event {
            n253 = event-data() -> ("ModuleID"=w301:i32, "Data"=w297:variant)  [unwired: 1 in]
            n254 = call <userlib>:"AddressedToThisModule.vi"("ModuleID"=w301, "ModuleAdmin"=w302) -> ("AddressedToThisInstance?"=w300:bool)  [unwired: 8 in, 1 out]
            n255 = case shown="True" w300 {
              tunnel: [_ w303] -> w299
              tunnel: w298 -> [_ w306]
              tunnel: w297 -> [_ w304]
              frame False {
              }
              frame True {
                n256 = call "Enqueue.vi"("Message Data"=w304, "Message"="ConfigTriggers", "MessageQueue"=w306) -> ("error out"=w303:errorcluster)  [unwired: 7 in, 1 out]
              }
            }
          }
          event User Event {
            n257 = event-data() -> ("ModuleID"=w311:i32, "Data"=w307:variant)  [unwired: 1 in]
            n258 = call <userlib>:"AddressedToThisModule.vi"("ModuleID"=w311, "ModuleAdmin"=w312) -> ("AddressedToThisInstance?"=w310:bool)  [unwired: 8 in, 1 out]
            n259 = case shown="True" w310 {
              tunnel: [_ w313] -> w309
              tunnel: w308 -> [_ w316]
              tunnel: w307 -> [_ w314]
              frame False {
              }
              frame True {
                n260 = call "Enqueue.vi"("Message Data"=w314, "Message"="Close", "MessageQueue"=w316) -> ("error out"=w313:errorcluster)  [unwired: 7 in, 1 out]
              }
            }
          }
        }
        n261 = call "ErrorHandler.vi"("error in (no error)"=w43, "MessageQueue"=w41) -> ("error out"=w42:errorcluster)  [unwired: 8 in, 1 out]
      }
    }
    frame Error {
      n262 = property class="ModuleAdmin.lvclass"(reference=w759) -> (reference out=w757:refnum<class "ModuleAdmin.lvclass">, "Accessors:CloneRegRef"=w756:refnum<data-value>, "Accessors:Module ID"=w755:i32)  [unwired: 1 in, 1 out]
      n263 = call <userlib>:"Remove.vi"("Module ID"=w755, "CloneRegRef"=w756) -> ("error out"=w760:errorcluster)  [unwired: 7 in, 2 out]
      n264 = flat-sequence {
        tunnel: w761 -> [w764]
        tunnel: w760 -> [_]
        tunnel: [w762] -> w753
        frame #0 {
          w763 = T12 2 items=["no dialog", "OK message", "continue or stop message", "OK message + warnings", "continue/stop + warnings"] ("type of dialog (OK msg:1)")
          n265 = call <vilib>:"Simple Error Handler.vi"("type of dialog (OK msg:1)"=w763, "error in (no error)"=w764) -> ("error out"=w762:errorcluster)  [unwired: 3 in, 4 out]
        }
      }
    }
  }
  n266 = call "DestroyClone.vi"("error in (no error)"=w13, "Exit via Stop Module Req?"=w9, "Wait for Module to stop?"=w10, "ModuleAdmin"=w11) -> ("error out"=w12:errorcluster, "External Launch"=w8:bool)  [unwired: 5 in, 1 out]
  n267 = Unregister For Events(event registration refnum=w3, error in=w4) -> (error out=w1:errorcluster)
  n268 = Release Queue(queue=w19, error in (no error)=w12) -> (error out=w7:errorcluster)  [unwired: 1 in, 2 out]
  n269 = Merge Errors(w1, w7) -> (w2:errorcluster)
  "error out" <- w2
  n270 = case shown="True" w8 {
    tunnel: w2 -> [_ w766]
    frame False {
    }
    frame True {
      n271 = control-ref of="This VI"() -> (w765:refnum<vi>)
      n272 = case shown="Error" w766 {
        tunnel: w765 -> [w767 w768]
        frame No Error {
          n273 = invoke class="VI" method="FP.Close"(reference=w767) -> ()  [unwired: 2 in, 3 out]
        }
        frame Error {
          n274 = invoke class="VI" method="FP.Open"(reference=w768, "Activate"=TRUE ("Activate?")) -> ()  [unwired: 3 in, 5 out]
        }
      }
    }
  }
